vi "Global 2.vi"() -> ()   [LabVIEW 2017]
panel:
  out "Boolean":bool=TRUE
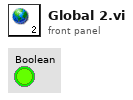
[diagram p1: front panel]
diagram:
